vi "szybka rejestracja - v2.vi"() -> ()   [LabVIEW 2009]
doc: "Use this template to build a producer/consumer design pattern. Use this template when you need to execute a process, such as data analysis, when a data source, such as a triggered acquisition, produces data at an uneven rate and you need to execute the process when the data becomes available."
uses:
  <vilib>/vision/Image Controls.llb/IMAQ Image.ctl
  Windows/System32/kernel32.dll
panel:
  out "Godzina/Time":string="09.12.02"
  in  "Rejest./Aqusit.":bool
  out "%RAM":u32(slide)=15 step=284519576 scale=0.0..100.0
  out "Nr zdj.(Pic No)":i32
  out "Image Out":T1(plugin-control)
  out "Elements in queue":i32
  in  "Frame/second":u8(ring) items=["1", "2", "5", "10", "50", "100", "200", "250", "333", "500", "1000"]
  in  "Number of buffers":u32=10
  in  "Region of interest":i32[](array[numeric])=[0, 0, 1280, 1024]
  in  "stop":bool
  # "Left"
  # "Top"
  # "Right"
  # "Bottom"
  # "OFF"
  # "ON"
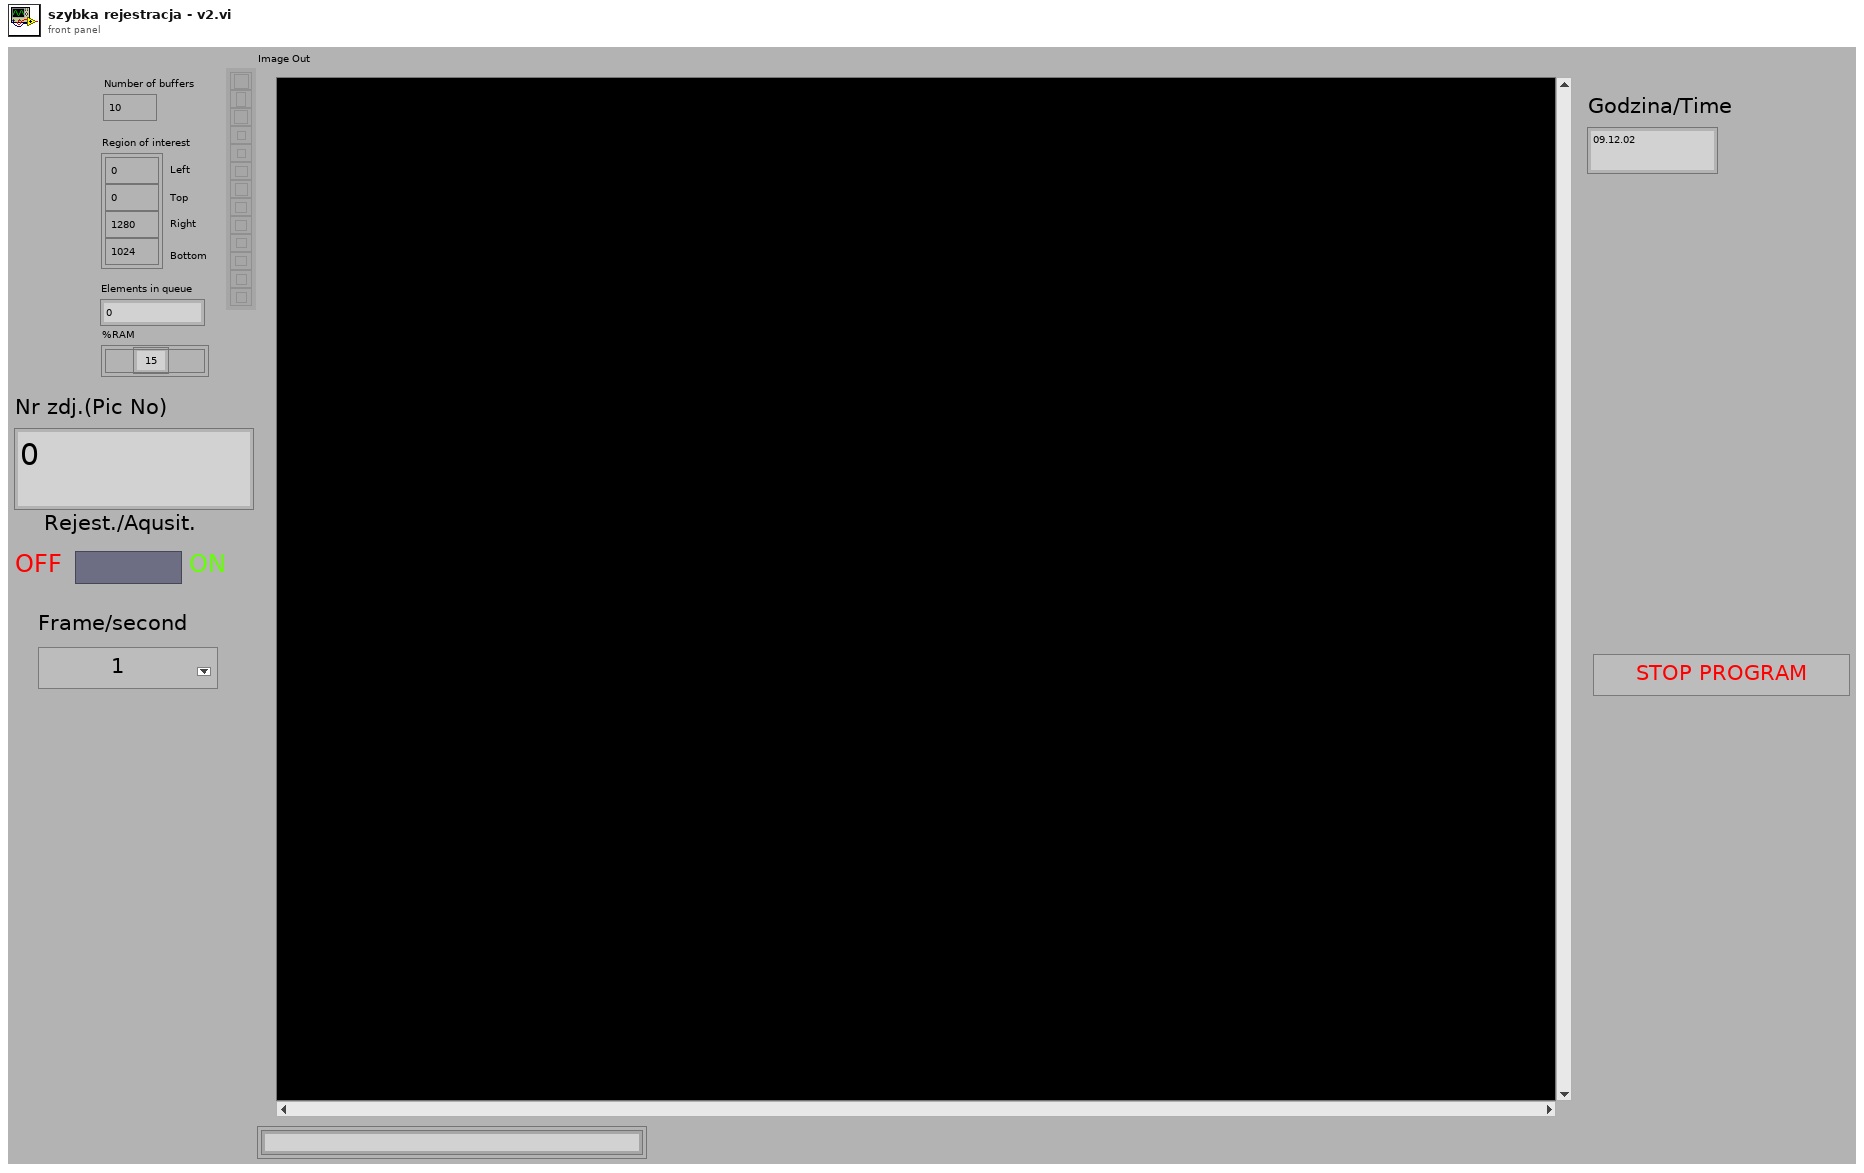
[diagram p1: front panel]
types:
  T1 = typedef "IMAQ Image.ctl" = refnum<image>
  T2 = cluster{"dwLength":u32, "dwMemoryLoad":u32, "dwTotalPhys":u32, "dwAvailPhys":u32, "dwTotalPageFile":u32, "dwAvailPageFile":u32, "dwTotalVirtual":u32, "dwAvailVirtual":u32}
  T3 = cluster{"New Image":T1, "czas":timestamp, "numer":i32, "fps":string}
  T4 = enum8{"Enabled", "Disabled", "Disabled and Grayed Out"}
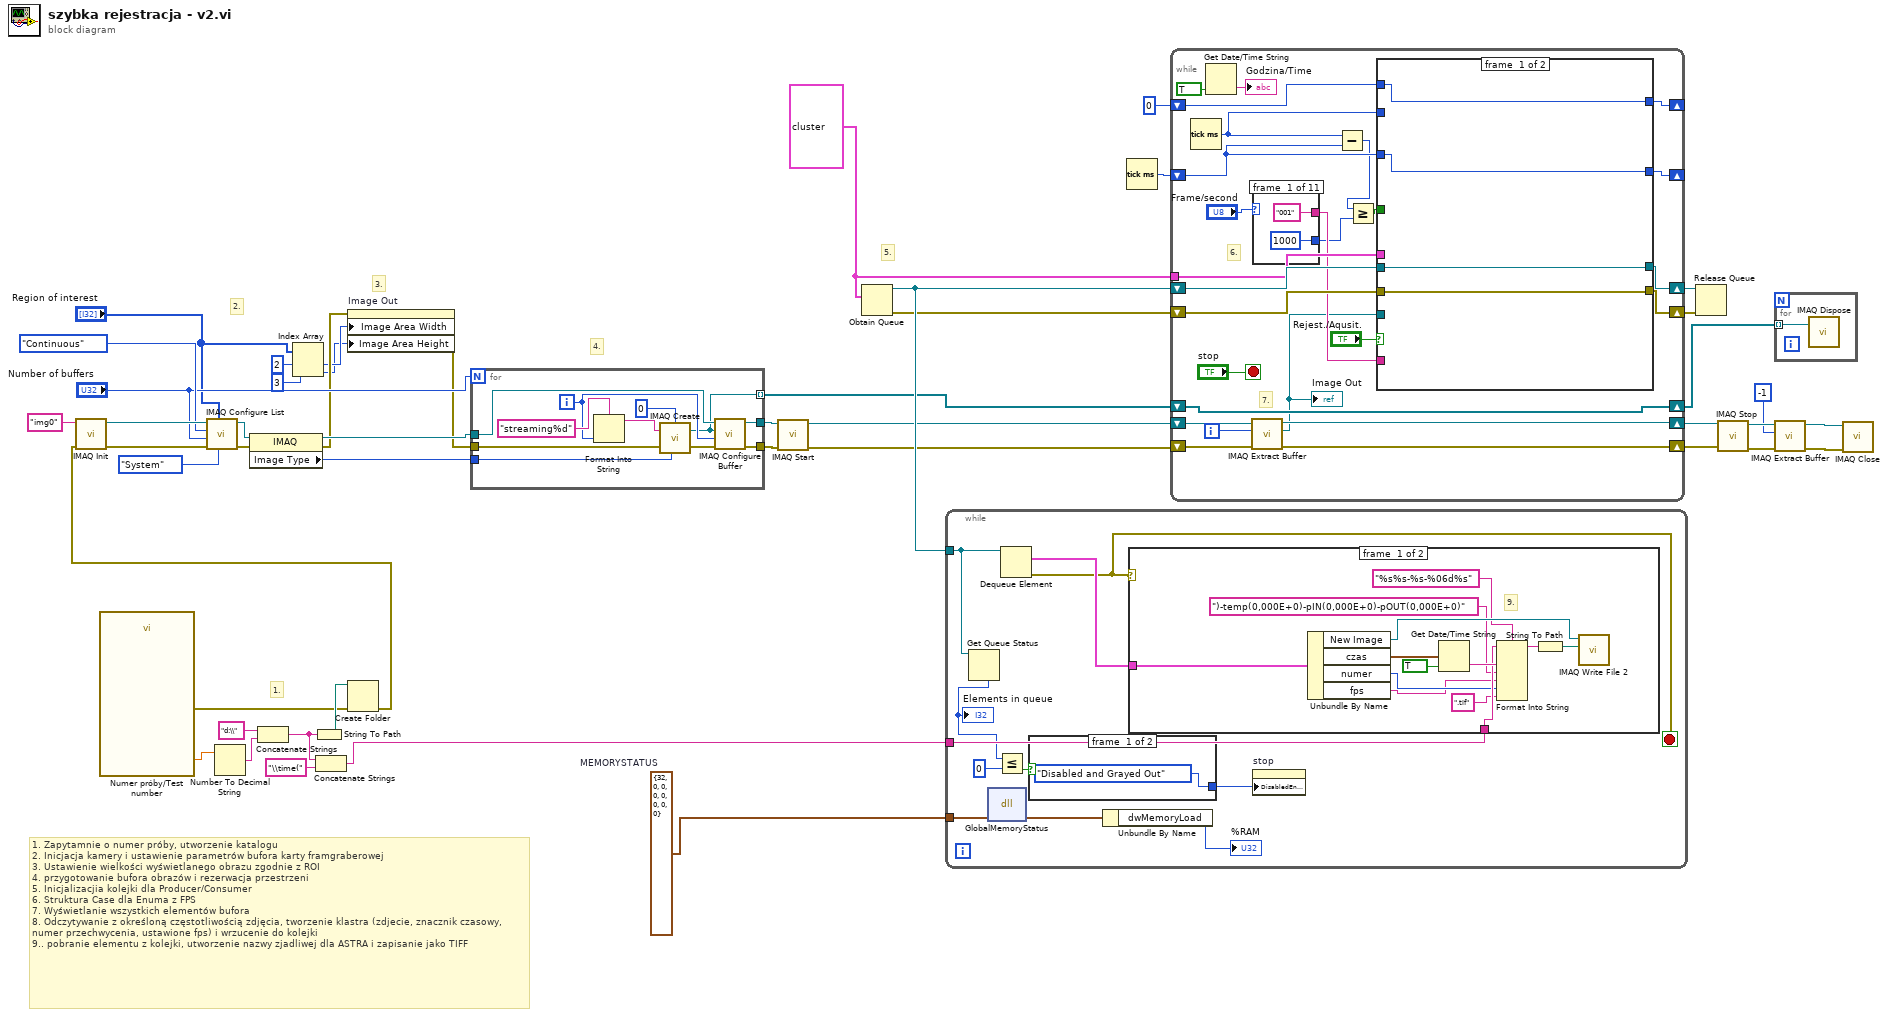
[diagram p0: block diagram]
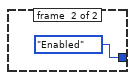
[diagram p2: hidden frame]
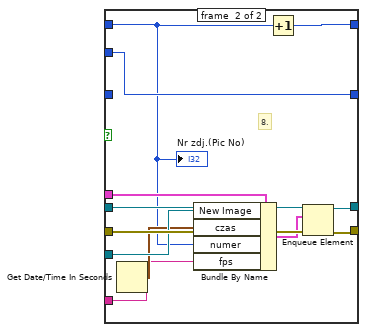
[diagram p5: hidden frame]
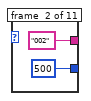
[diagram p6: hidden frame]
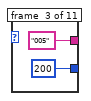
[diagram p7: hidden frame]
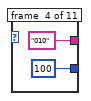
[diagram p8: hidden frame]
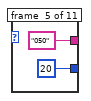
[diagram p9: hidden frame]
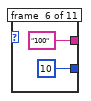
[diagram p10: hidden frame]
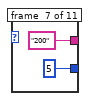
[diagram p11: hidden frame]
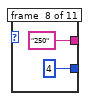
[diagram p12: hidden frame]
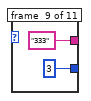
[diagram p13: hidden frame]
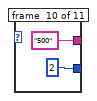
[diagram p14: hidden frame]
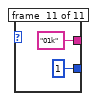
[diagram p15: hidden frame]
diagram:
  w1 = T2 {"dwLength"=32, "dwMemoryLoad"=0, "dwTotalPhys"=0, "dwAvailPhys"=0, "dwTotalPageFile"=0, "dwAvailPageFile"=0, "dwTotalVirtual"=0, "dwAvailVirtual"=0}  # MEMORYSTATUS
  w27 = T3 data[76B]
  # "1. Zapytamnie o numer próby, utworzenie katalogu\n2. Inicjacja kamery i ustawienie parametrów bufora karty framgraberowej\n3. Ustawienie wielkości wyświetlanego obrazu zgodnie z ROI\n4. przygotowanie bufora obrazów i rezerwacja przestrzeni\n5. Inicjalizacjia kolejki dla Producer/Consumer\n6. Struktura Case dla Enuma z FPS\n7. Wyświetlanie wszystkich elementów bufora\n8. Odczytywanie z określoną częstotliwością zdjęcia, tworzenie klastra (zdjecie, znacznik czasowy, numer przechwycenia, ustawione fps) i wrzucenie do kolejki\n9.. pobranie elementu z kolejki, utworzenie nazwy zjadliwej dla ASTRA i zapisanie jako TIFF"
  # "5."
  # "4."
  # "3."
  # "2."
  # "1."
  n1 = call "Numer próby/Test number"() -> ("Numer próby"=w7:dbl, "error out"=w6:errorcluster)  [unwired: 17 in, 1 out]
  n2 = Number To Decimal String(number=w7) -> (decimal integer string=w8:string)  [unwired: 1 in]
  n3 = Concatenate Strings("d:\\", w8) -> (w4:string)
  n4 = Index Array(array="Region of interest", index #1=2 ("index"), index #2=3 ("index")) -> (element #1=w12:i32, element #2=w11:i32)
  n5 = String To Path(string=w4) -> (path=w10:path)
  n6 = Concatenate Strings(w4, "\\time(" ("string")) -> (w2:string)
  n7 = Create Folder(path (use dialog)=w10, error in=w6) -> (error out=w5:errorcluster)  [unwired: 1 in, 2 out]
  n8 = call <vilib>:"IMAQ Init.vi"("error in (no error)"=w5, "Interface Name"="img0") -> ("error out"=w40:errorcluster, "IMAQ Session Out"=w39:refnum<k11>)  [unwired: 8 in]
  n9 = call <vilib>:"IMAQ Configure List.vi"("Memory Location"=enum16{"System", "Onboard"}."System", "Region of interest"="Region of interest", "error in (no error)"=w40, "Number of buffers"="Number of buffers", "Continuous?"=enum16{"One-Shot", "Continuous"}."Continuous", "IMAQ Session In"=w39) -> ("error out"=w35:errorcluster, "IMAQ Session Out"=w36:refnum<k11>)  [unwired: 4 in]
  n10 = property class="IMAQ"(reference=w36, error in=w35) -> (reference out=w33:refnum<k11>, error out=w17:errorcluster, "Image Type"=w32:u32)
  n11 = property on="Image Out" class="ImageControl"(error in=w17, "Image Area Width"=w12, "Image Area Height"=w11) -> (error out=w16:errorcluster)  [unwired: 1 in, 1 out]
  n12 = for {
    N: "Number of buffers" -> [_]
    tunnel: w33 -> [w54]
    tunnel: w16 -> [w56]
    tunnel: w32 -> [w58]
    tunnel: [w50] -> w30
    tunnel: [w49] -> w31
    tunnel: [w48] -> w19 mode=indexing
    i -> [w51]
    n13 = Format Into String(format string="streaming%d", w51) -> (resulting string=w52:string)  [unwired: 2 in, 1 out]
    n14 = call "IMAQ Create"("Border Size"=0, "Image Name"=w52, "Image Type"=w58, "error in (no error)"=w56) -> ("New Image"=w48:T1, "error out"=w53:errorcluster)  [unwired: 1 in]
    n15 = call <vilib>:"IMAQ Configure Buffer.vi"("error in (no error)"=w53, "Buffer Number"=w51, "Image In"=w48, "IMAQ Session In"=w54) -> ("error out"=w49:errorcluster, "IMAQ Session Out"=w50:refnum<k11>)  [unwired: 6 in]
  }
  n16 = call <vilib>:"IMAQ Start.vi"("error in (no error)"=w31, "IMAQ Session In"=w30) -> ("error out"=w28:errorcluster, "IMAQ Session Out"=w29:refnum<k11>)  [unwired: 8 in]
  n17 = Obtain Queue(element data type=w27) -> (queue out=w47:refnum<queue>, error out=w46:errorcluster)  [unwired: 4 in, 1 out]
  n18 = while {
    tunnel: w47 -> [w68]
    tunnel: w2 -> [w67]
    tunnel: w1 -> [w65]
    stop <- w66 stop-if-true
    n19 = Get Queue Status(queue=w68) -> (# elements in queue=w62:i32)  [unwired: 2 in, 7 out]
    "Elements in queue" <- w62
    n20 = dll-call lib="C:/Windows/System32/Kernel32.dll" fn="GlobalMemoryStatus"("lpMemoryStatus"=w65) -> ("lpMemoryStatus"=w64:T2)  [unwired: 4 in, 2 out]
    n21 = Less Or Equal?(x=w62, y=0) -> (x <= y?=w59:bool)
    n22 = Dequeue Element(queue=w68) -> (element=w69:T3, error out=w66:errorcluster)  [unwired: 2 in, 2 out]
    n23 = case shown="False" w59 {
      tunnel: [T4."Disabled and Grayed Out" ("Disabled") T4."Enabled" ("Disabled")] -> w60
      frame #0 {
      }
      frame #1 {
      }
    }
    n24 = Unbundle By Name(w64) -> ("dwMemoryLoad"=→"%RAM":u32)
    n25 = case shown="No Error" w66 {
      tunnel: w69 -> [w78 _]
      tunnel: w67 -> [w76 _]
      frame #0 {
        # "9."
        n26 = Unbundle By Name(w78) -> ("New Image"=w84:T1, "czas"=w81:timestamp, "numer"=w73:i32, "fps"=w72:string)
        n27 = Get Date/Time String(seconds (now)=w81, want seconds? (F)=TRUE) -> (time string=w80:string)  [unwired: 1 in, 1 out]
        n28 = Format Into String(format string="%s%s-%s-%06d%s", initial string=w76, w80, ")-temp(0,000E+0)-pIN(0,000E+0)-pOUT(0,000E+0)" ("string"), w72, w73, ".tif") -> (resulting string=w83:string)  [unwired: 1 in, 1 out]
        n29 = String To Path(string=w83) -> (path=w82:path)
        n30 = call-poly "IMAQ Write File 2"("File Path"=w82, "Image"=w84) -> ()  [unwired: 8 in, 2 out]
      }
      frame #1 {
      }
    }
    n31 = property on="stop" class="Bool"("DisabledEnum"=w60) -> ()  [unwired: 2 in, 2 out]
  }
  n32 = Tick Count (ms)() -> (millisecond timer value=w43:u32)
  n33 = while {
    shift-right: [w106] -> w44
    shift-left: w46 -> [w107]
    shift-right: [w108] -> w45
    shift-left: w47 -> [w109]
    shift-right: [w100] -> _
    shift-left: w43 -> [w104]
    shift-right: [w101] -> _
    shift-left: 0 -> [w102]
    tunnel: w27 -> [w96]
    shift-right: [w95] -> w22
    shift-left: w29 -> [w99]
    shift-right: [w94] -> w21
    shift-left: w28 -> [w98]
    shift-right: [w90] -> w18
    shift-left: w19 -> [w90]
    i -> [w97]
    stop <- "stop" stop-if-true
    # "7."
    # "6."
    n34 = Tick Count (ms)() -> (millisecond timer value=w105:u32)
    n35 = Get Date/Time String(want seconds? (F)=TRUE) -> (time string=→"Godzina/Time":string)  [unwired: 2 in, 1 out]
    n36 = call <vilib>:"IMAQ Extract Buffer.vi"("error in (no error)"=w98, "Buffer to extract"=w97, "IMAQ Session In"=w99) -> ("error out"=w94:errorcluster, "Image Out"=w89:T1, "IMAQ Session Out"=w95:refnum<k11>)  [unwired: 3 in, 3 out]
    "Image Out" <- w89
    n37 = case shown="2" "Frame/second" {
      tunnel: [1000 500 200 100 20 10 5 4 3 2 1] -> w91
      tunnel: ["001" "002" "005" "010" "050" "100" "200" "250" "333" "500" "01k"] -> w92
      frame #0 {
      }
      frame #1 {
      }
      frame #2 {
      }
      frame #3 {
      }
      frame #4 {
      }
      frame #5 {
      }
      frame #6 {
      }
      frame #7 {
      }
      frame #8 {
      }
      frame #9 {
      }
      frame #10 {
      }
    }
    n38 = Subtract(x=w105, y=w104) -> (x-y=w88:u32)
    n39 = Greater Or Equal?(x=w88, y=w91) -> (x >= y?=w103:bool)
    n40 = case shown="False" "Rejest./Aqusit." {
      tunnel: w109 -> [w112 w127]
      tunnel: [w112 w126] -> w108
      tunnel: w107 -> [w111 w125]
      tunnel: [w111 w124] -> w106
      tunnel: w105 -> [_ w123]
      tunnel: w104 -> [w113 w122]
      tunnel: w103 -> [_ w121]
      tunnel: w102 -> [w114 w120]
      tunnel: [w114 w119] -> w101
      tunnel: [w113 w118] -> w100
      tunnel: w96 -> [_ w117]
      tunnel: w92 -> [_ w116]
      tunnel: w89 -> [_ w115]
      frame #0 {
      }
      frame #1 {
        n41 = case shown="True" w121 {
          tunnel: w127 -> [w131 w143]
          tunnel: [w131 w142] -> w126
          tunnel: w125 -> [w130 w141]
          tunnel: [w130 w140] -> w124
          tunnel: w123 -> [_ w138]
          tunnel: w122 -> [w128 _]
          tunnel: w120 -> [w129 w134]
          tunnel: [w129 w139] -> w119
          tunnel: [w128 w138] -> w118
          tunnel: w115 -> [_ w136]
          tunnel: w117 -> [_ w137]
          tunnel: w116 -> [_ w132]
          frame #0 {
          }
          frame #1 {
            # "8."
            n42 = Get Date/Time In Seconds() -> (seconds since 1Jan1904=w135:timestamp)
            n43 = Bundle By Name(cluster=w137, "New Image"=w136, "czas"=w135, "numer"=w134, "fps"=w132) -> (w133:T3)
            n44 = Increment(x=w134) -> (x+1=w139:i32)
            n45 = Enqueue Element(queue=w143, element=w133, error in (no error)=w141) -> (queue out=w142:refnum<queue>, error out=w140:errorcluster)  [unwired: 1 in, 1 out]
            "Nr zdj.(Pic No)" <- w134
          }
        }
      }
    }
  }
  n46 = Release Queue(queue=w45, error in (no error)=w44) -> ()  [unwired: 1 in, 3 out]
  n47 = call <vilib>:"IMAQ Stop.vi"("error in (no error)"=w21, "IMAQ Session In"=w22) -> ("error out"=w24:errorcluster, "IMAQ Session Out"=w23:refnum<k11>)  [unwired: 8 in]
  n48 = for {
    tunnel: w18 -> [w166] mode=indexing
    n49 = call "IMAQ Dispose"("Image"=w166) -> ()  [unwired: 5 in, 1 out]
  }
  n50 = call <vilib>:"IMAQ Extract Buffer.vi"("error in (no error)"=w24, "Buffer to extract"=-1, "IMAQ Session In"=w23) -> ("error out"=w25:errorcluster, "IMAQ Session Out"=w26:refnum<k11>)  [unwired: 3 in, 4 out]
  n51 = call <vilib>:"IMAQ Close.vi"("error in (no error)"=w25, "IMAQ Session In"=w26) -> ()  [unwired: 9 in, 1 out]
